vi "LV8_5.vi"() -> ()   [LabVIEW 2016]
uses:
  <vilib>/sound2/lvsound2.llb/Sampling Mode.ctl
  <vilib>/sound2/lvsound2.llb/Sound Output Write (DBL Single).vi
  <vilib>/Utility/file.llb/Read From Spreadsheet File (DBL).vi
panel:
  in  "radius of poles":dbl(slide)=0.99 scale=0.1..0.99
  in  "fundamental frequency":dbl(slide)=436.0 scale=400.0..500.0
  out "Filtered signal (freq domain)":cluster{"F":dbl[], "FYI":dbl[]}(graph)
  out "Original signal (freq domain)":cluster{"W":dbl[], "H":dbl[]}[](graph)
  out "Original signal (time domain)":cluster{"t":dbl[], "first row":dbl[]}(graph)={"t"=[0.022675736961451247, 0.022698412698412697, 0.02272108843537415, 0.0227437641723356, 0.022766439909297054, 0.022789115646258504, 0.022811791383219954, 0.022834467120181407, 0.022857142857142857, 0.022879818594104307, 0.02290249433106576, 0.02292517006802721, 0.02294784580498866, 0.022970521541950114, 0.022993197278911564, 0.023015873015873017, 0.023038548752834467, 0.023061224489795917, 0.02308390022675737, 0.02310657596371882, 0.02312925170068027, 0.023151927437641724, 0.023174603174603174, 0.023197278911564624, 0.023219954648526078, 0.023242630385487528, 0.02326530612244898, 0.02328798185941043, 0.02331065759637188, 0.023333333333333334, 0.023356009070294784, 0.023378684807256234, 0.023401360544217688, 0.023424036281179138, 0.02344671201814059, 0.02346938775510204, 0.02349206349206349, 0.023514739229024945, 0.023537414965986395, 0.023560090702947845, 0.023582766439909298, 0.023605442176870748, 0.023628117913832198, 0.02365079365079365, 0.0236734693877551, 0.023696145124716555, 0.023718820861678005, 0.023741496598639455, 0.023764172335600908, 0.023786848072562358, 0.023809523809523808, 0.02383219954648526, 0.02385487528344671, 0.02387755102040816, 0.023900226757369615, 0.023922902494331065, 0.02394557823129252, 0.02396825396825397, 0.02399092970521542, 0.024013605442176872, 0.024036281179138322, 0.024058956916099772, 0.024081632653061225, 0.024104308390022675, 0.02412698412698413, 0.02414965986394558, 0.02417233560090703, 0.024195011337868482, 0.024217687074829932, 0.024240362811791382, 0.024263038548752835, 0.024285714285714285, 0.024308390022675735, 0.02433106575963719, 0.02435374149659864, 0.024376417233560092, 0.024399092970521542, 0.024421768707482992, 0.024444444444444446, 0.024467120181405896, 0.024489795918367346, 0.0245124716553288, 0.02453514739229025, 0.0245578231292517, 0.024580498866213153, 0.024603174603174603, 0.024625850340136056, 0.024648526077097506, 0.024671201814058956, 0.02469387755102041, 0.02471655328798186, 0.02473922902494331, 0.024761904761904763, 0.024784580498866213, 0.024807256235827663, 0.024829931972789116, 0.024852607709750566, 0.02487528344671202, 0.02489795918367347, 0.02492063492063492, 0.024943310657596373, 0.024965986394557823, 0.024988662131519273, 0.025011337868480726, 0.025034013605442176, 0.02505668934240363, 0.02507936507936508, 0.02510204081632653, 0.025124716553287983, 0.025147392290249433, 0.025170068027210883, 0.025192743764172337, 0.025215419501133787, 0.025238095238095237, 0.02526077097505669, 0.02528344671201814, 0.025306122448979593, 0.025328798185941043, 0.025351473922902493, 0.025374149659863947, 0.025396825396825397, 0.025419501133786847, 0.0254421768707483, 0.02546485260770975, 0.0254875283446712, 0.025510204081632654, 0.025532879818594104, 0.025555555555555557, 0.025578231292517007, 0.025600907029478457, 0.02562358276643991, 0.02564625850340136, 0.02566893424036281, 0.025691609977324264, 0.025714285714285714, 0.025736961451247164, 0.025759637188208617, 0.025782312925170067, 0.02580498866213152, 0.02582766439909297, 0.02585034013605442, 0.025873015873015874, 0.025895691609977324, 0.025918367346938774, 0.025941043083900227, 0.025963718820861677, 0.02598639455782313, 0.02600907029478458, 0.02603174603174603, 0.026054421768707484, 0.026077097505668934, 0.026099773242630384, 0.026122448979591838, 0.026145124716553288, 0.026167800453514738, 0.02619047619047619, 0.02621315192743764, 0.026235827664399095, 0.026258503401360545, 0.026281179138321994, 0.026303854875283448, 0.026326530612244898, 0.026349206349206348, 0.0263718820861678, 0.02639455782312925, 0.0264172335600907, 0.026439909297052155, 0.026462585034013605, 0.026485260770975058, 0.026507936507936508, 0.026530612244897958, 0.02655328798185941, 0.02657596371882086, 0.02659863945578231, 0.026621315192743765, 0.026643990929705215, 0.02666666666666667, 0.02668934240362812, 0.02671201814058957, 0.026734693877551022, 0.026757369614512472, 0.02678004535147392, 0.026802721088435375, 0.026825396825396825, 0.026848072562358275, 0.02687074829931973, 0.02689342403628118, 0.026916099773242632, 0.026938775510204082, 0.026961451247165532, 0.026984126984126985, 0.027006802721088435, 0.027029478458049885, 0.02705215419501134, 0.02707482993197279, 0.02709750566893424, 0.027120181405895692, 0.027142857142857142, 0.027165532879818596, 0.027188208616780046], "first row"=array[32768 elements]}
  out "Filtered signal (time domain)":cluster{"t":dbl[], "Y":dbl[]}(graph)={"t"=[0.022675736961451247, 0.022698412698412697, 0.02272108843537415, 0.0227437641723356, 0.022766439909297054, 0.022789115646258504, 0.022811791383219954, 0.022834467120181407, 0.022857142857142857, 0.022879818594104307, 0.02290249433106576, 0.02292517006802721, 0.02294784580498866, 0.022970521541950114, 0.022993197278911564, 0.023015873015873017, 0.023038548752834467, 0.023061224489795917, 0.02308390022675737, 0.02310657596371882, 0.02312925170068027, 0.023151927437641724, 0.023174603174603174, 0.023197278911564624, 0.023219954648526078, 0.023242630385487528, 0.02326530612244898, 0.02328798185941043, 0.02331065759637188, 0.023333333333333334, 0.023356009070294784, 0.023378684807256234, 0.023401360544217688, 0.023424036281179138, 0.02344671201814059, 0.02346938775510204, 0.02349206349206349, 0.023514739229024945, 0.023537414965986395, 0.023560090702947845, 0.023582766439909298, 0.023605442176870748, 0.023628117913832198, 0.02365079365079365, 0.0236734693877551, 0.023696145124716555, 0.023718820861678005, 0.023741496598639455, 0.023764172335600908, 0.023786848072562358, 0.023809523809523808, 0.02383219954648526, 0.02385487528344671, 0.02387755102040816, 0.023900226757369615, 0.023922902494331065, 0.02394557823129252, 0.02396825396825397, 0.02399092970521542, 0.024013605442176872, 0.024036281179138322, 0.024058956916099772, 0.024081632653061225, 0.024104308390022675, 0.02412698412698413, 0.02414965986394558, 0.02417233560090703, 0.024195011337868482, 0.024217687074829932, 0.024240362811791382, 0.024263038548752835, 0.024285714285714285, 0.024308390022675735, 0.02433106575963719, 0.02435374149659864, 0.024376417233560092, 0.024399092970521542, 0.024421768707482992, 0.024444444444444446, 0.024467120181405896, 0.024489795918367346, 0.0245124716553288, 0.02453514739229025, 0.0245578231292517, 0.024580498866213153, 0.024603174603174603, 0.024625850340136056, 0.024648526077097506, 0.024671201814058956, 0.02469387755102041, 0.02471655328798186, 0.02473922902494331, 0.024761904761904763, 0.024784580498866213, 0.024807256235827663, 0.024829931972789116, 0.024852607709750566, 0.02487528344671202, 0.02489795918367347, 0.02492063492063492, 0.024943310657596373, 0.024965986394557823, 0.024988662131519273, 0.025011337868480726, 0.025034013605442176, 0.02505668934240363, 0.02507936507936508, 0.02510204081632653, 0.025124716553287983, 0.025147392290249433, 0.025170068027210883, 0.025192743764172337, 0.025215419501133787, 0.025238095238095237, 0.02526077097505669, 0.02528344671201814, 0.025306122448979593, 0.025328798185941043, 0.025351473922902493, 0.025374149659863947, 0.025396825396825397, 0.025419501133786847, 0.0254421768707483, 0.02546485260770975, 0.0254875283446712, 0.025510204081632654, 0.025532879818594104, 0.025555555555555557, 0.025578231292517007, 0.025600907029478457, 0.02562358276643991, 0.02564625850340136, 0.02566893424036281, 0.025691609977324264, 0.025714285714285714, 0.025736961451247164, 0.025759637188208617, 0.025782312925170067, 0.02580498866213152, 0.02582766439909297, 0.02585034013605442, 0.025873015873015874, 0.025895691609977324, 0.025918367346938774, 0.025941043083900227, 0.025963718820861677, 0.02598639455782313, 0.02600907029478458, 0.02603174603174603, 0.026054421768707484, 0.026077097505668934, 0.026099773242630384, 0.026122448979591838, 0.026145124716553288, 0.026167800453514738, 0.02619047619047619, 0.02621315192743764, 0.026235827664399095, 0.026258503401360545, 0.026281179138321994, 0.026303854875283448, 0.026326530612244898, 0.026349206349206348, 0.0263718820861678, 0.02639455782312925, 0.0264172335600907, 0.026439909297052155, 0.026462585034013605, 0.026485260770975058, 0.026507936507936508, 0.026530612244897958, 0.02655328798185941, 0.02657596371882086, 0.02659863945578231, 0.026621315192743765, 0.026643990929705215, 0.02666666666666667, 0.02668934240362812, 0.02671201814058957, 0.026734693877551022, 0.026757369614512472, 0.02678004535147392, 0.026802721088435375, 0.026825396825396825, 0.026848072562358275, 0.02687074829931973, 0.02689342403628118, 0.026916099773242632, 0.026938775510204082, 0.026961451247165532, 0.026984126984126985, 0.027006802721088435, 0.027029478458049885, 0.02705215419501134, 0.02707482993197279, 0.02709750566893424, 0.027120181405895692, 0.027142857142857142, 0.027165532879818596, 0.027188208616780046], "Y"=array[32768 elements]}
  in  "Play original sound":bool
  in  "Play filtered sound":bool
  in  "stop":bool
  # "A note = 440 Hz"
  # "B note = 494 Hz"
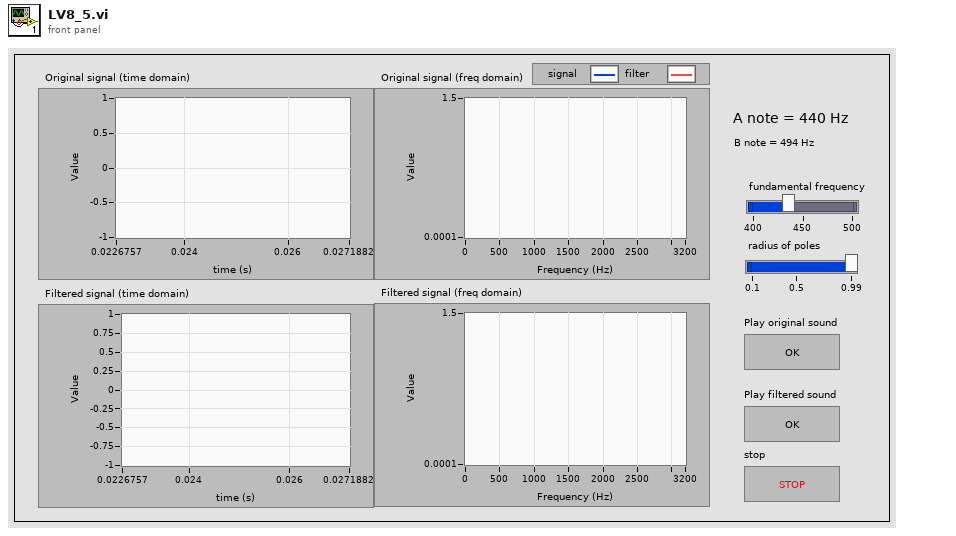
[diagram p1: front panel]
types:
  T1 = typedef "Sampling Mode.ctl" = i32
  T2 = typedef "Sound Output Task ID.ctl" = u32
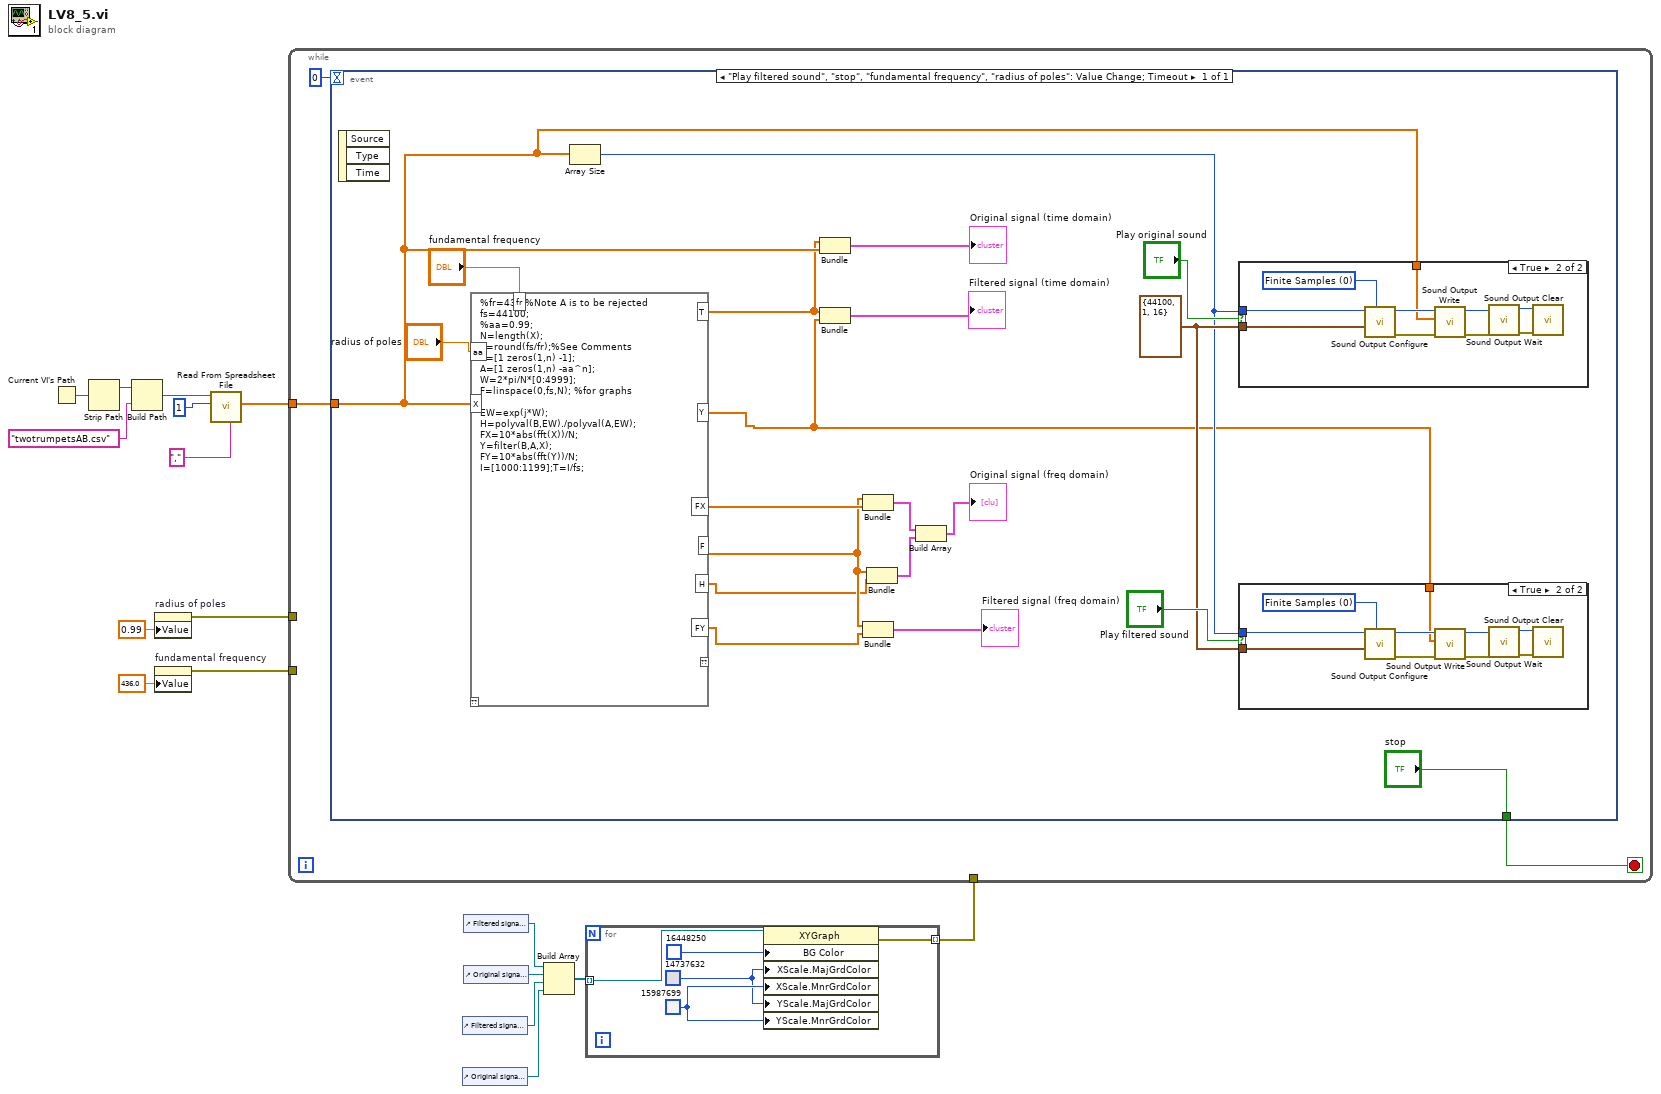
[diagram p0: block diagram]
diagram:
  n1 = Current VI's Path() -> (path=w17:path)
  n2 = Strip Path(path=w17) -> (stripped path=w16:path)  [unwired: 1 out]
  n3 = Build Path(base path=w16, name or relative path="twotrumpetsAB.csv") -> (appended path=w14:path)
  n4 = property on="radius of poles" class="Slide (strict)"("Value"=0.99 ("minus real part of poles")) -> (error out=w10:errorcluster)  [unwired: 2 in, 1 out]
  n5 = property on="fundamental frequency" class="Slide (strict)"("Value"=436.0 ("fundamental frequency")) -> (error out=w9:errorcluster)  [unwired: 2 in, 1 out]
  n6 = call-poly <vilib>:"Read From Spreadsheet File.vi"("delimiter (\\t)"="," ("delimiter (\\t)"), "number of rows (all:-1)"=1, "file path (dialog if empty)"=w14) -> ("first row"=w11:dbl[])  [unwired: 4 in, 4 out]
  n7 = control-ref of="Filtered signal (time domain)"() -> (w3:refnum<vi>)
  n8 = control-ref of="Original signal (freq domain)"() -> (w2:refnum<vi>)
  n9 = control-ref of="Filtered signal (freq domain)"() -> (w5:refnum<vi>)
  n10 = control-ref of="Original signal (time domain)"() -> (w4:refnum<vi>)
  n11 = Build Array(w5, w4, w3, w2) -> (w6:refnum<vi>[])
  n12 = for {
    tunnel: w6 -> [w19] mode=indexing
    tunnel: [w18] -> w1 mode=indexing
    w21 = u32 15987699
    w20 = u32 14737632
    n13 = property class="XYGraph"(reference=w19, "BG Color"=u32 16448250, "XScale.MajGrdColor"=w20, "XScale.MnrGrdColor"=w21, "YScale.MajGrdColor"=w20, "YScale.MnrGrdColor"=w21) -> (error out=w18:errorcluster)  [unwired: 1 in, 1 out]
  }
  n14 = while {
    tunnel: w11 -> [w25]
    tunnel: w10 -> [_]
    tunnel: w9 -> [_]
    tunnel: w1 -> [_]
    stop <- w24 stop-if-true
    n15 = event shown="[0] \"Play filtered sound\", \"stop\", \"fundamental frequency\", \"radius of poles\": Value Change;  Timeout" {
      selector: _ -> [_]
      dyn-events: _ -> [_]
      timeout: 0 -> [_]
      tunnel: w25 -> [w43]
      tunnel: ["stop"] -> w24
      event "Play filtered sound", "stop", "fundamental frequency", "radius of poles": Value Change; Timeout {
        w41 = cluster{"fs":i32, i32, i32} {"fs"=44100, 1, 16}
        n16 = event-data() -> ()  [unwired: 1 in, 3 out]
        n17 = mathscript code="%fr=436;%Note A is to be rejected\nfs=44100;\n%aa=0.99;\nN=length(X);\nn=round(fs/fr);%See Comments\nB=[1 zeros(1,n) -1];\nA=[1 zeros(1,n) -aa^n];\nW=2*pi/N*[0:4999];\nF=linspace(0,fs,N); %for graphs\n\nEW=exp(j*W);\nH=polyval(B,EW)./polyval(A,EW);\nFX=10*abs(fft(X))/N;\nY=filter(B,A,X);\nFY=10*abs(fft(Y))/N;\nI=[1000:1199];T=I/fs;"("X"=w43, "aa"="radius of poles", "fr"="fundamental frequency") -> ("Y"=w32:cdb[], "F"=w37:dbl[], "FY"=w30:dbl[], "T"=w34:dbl[], "FX"=w38:dbl[], "H"=w31:cdb[])  [unwired: 1 in, 1 out]
        n18 = Array Size(array=w43) -> (size(s)=w40:i32)
        n19 = Bundle("T"=w34, "first row"=w43) -> (→"Original signal (time domain)":cluster{"T":dbl[], "first row":dbl[]})  [unwired: 1 in]
        n20 = Bundle("T"=w34, "Y"=w32) -> (→"Filtered signal (time domain)":cluster{"T":dbl[], "Y":cdb[]})  [unwired: 1 in]
        n21 = Bundle("F"=w37, "FX"=w38) -> (w28:cluster{"F":dbl[], "FX":dbl[]})  [unwired: 1 in]
        n22 = Bundle("F"=w37, "FY"=w30) -> (→"Filtered signal (freq domain)":cluster{"F":dbl[], "FY":dbl[]})  [unwired: 1 in]
        n23 = Bundle("F"=w37, "H"=w31) -> (w27:cluster{"F":dbl[], "H":cdb[]})  [unwired: 1 in]
        n24 = Build Array(w28, w27) -> (→"Original signal (freq domain)":cluster{"F":dbl[], "H":cdb[]}[])
        n25 = case shown="True" "Play original sound" {
          tunnel: w41 -> [_ w59]
          tunnel: w40 -> [_ w57]
          tunnel: w43 -> [_ w56]
          frame False {
          }
          frame True {
            w58 = T1 0 items=["Finite Samples", "Continuous Samples"] ("sample mode")
            n26 = call <vilib>:"Sound Output Configure.vi"("number of samples/ch"=w57, "sample mode"=w58, "sound format"=w59) -> ("error out"=w60:errorcluster, "task ID"=w65:T2)  [unwired: 7 in]
            n27 = call-poly <vilib>:"Sound Output Write.vi"("error in (no error)"=w60, "data"=w56, "task ID"=w65) -> ("error out"=w61:errorcluster, "task ID out"=w62:T2)  [unwired: 7 in]
            n28 = call <vilib>:"Sound Output Wait.vi"("error in (no error)"=w61, "task ID"=w62) -> ("error out"=w64:errorcluster, "task ID out"=w63:T2)  [unwired: 8 in]
            n29 = call <vilib>:"Sound Output Clear.vi"("error in (no error)"=w64, "task ID"=w63) -> ()  [unwired: 9 in, 1 out]
          }
        }
        n30 = case shown="True" "Play filtered sound" {
          tunnel: w41 -> [_ w49]
          tunnel: w40 -> [_ w47]
          tunnel: w32 -> [_ w46]
          frame False {
          }
          frame True {
            w48 = T1 0 items=["Finite Samples", "Continuous Samples"] ("sample mode")
            n31 = call <vilib>:"Sound Output Configure.vi"("number of samples/ch"=w47, "sample mode"=w48, "sound format"=w49) -> ("error out"=w50:errorcluster, "task ID"=w55:T2)  [unwired: 7 in]
            n32 = call-poly <vilib>:"Sound Output Write.vi"("error in (no error)"=w50, "data"=w46, "task ID"=w55) -> ("error out"=w51:errorcluster, "task ID out"=w52:T2)  [unwired: 7 in]
            n33 = call <vilib>:"Sound Output Wait.vi"("error in (no error)"=w51, "task ID"=w52) -> ("error out"=w54:errorcluster, "task ID out"=w53:T2)  [unwired: 8 in]
            n34 = call <vilib>:"Sound Output Clear.vi"("error in (no error)"=w54, "task ID"=w53) -> ()  [unwired: 9 in, 1 out]
          }
        }
      }
    }
  }
